vi "MenySMO.vi"() -> ()   [LabVIEW 2018]
uses:
  <vilib>/addons/database/Connection.llb/Conn ObjectReference.ctl
  <vilib>/addons/database/Connection.llb/DB Tools Open Connec (Path).vi
  <vilib>/addons/database/NI_Database_API.lvlib
panel:
  out "Menu Home":bool
  out "Menu Suma":bool
  out "Menu Precios":bool
  in  "Menu":enum32{"Venta", "Precios", "Precios 2"}(tab)
  in  "Guardar Orden":bool
  in  "Reiniciar Orden":bool
  out "Cambio (Pesos)":dbl
  out "TOTAL":dbl
  in  "Orden":string
  in  "PAGO CON:":dbl
  out "Dolares":bool
  out "Tarjeta":bool
  out "Pesos":bool=TRUE
  out "Producto 6":bool
  out "Producto 5":bool
  out "Producto 4":bool
  out "Producto 3":bool
  out "Producto 2":bool
  out "Producto 1":bool
  in  "Tipo de Cambio Dolares":dbl=19.0
  in  "Precio ARROZ CON LECHE":dbl=30.0
  in  "Precio BANDERILLA":dbl=50.0
  in  "Precio PAPAS LOCAS":dbl=50.0
  in  "Precio GOMITAS":dbl=35.0
  in  "Precio PAY DE QUESO":dbl=35.0
  in  "Precio PAN DE MUERTO":dbl=70.0
  in  "Productos":i32(listbox)
  in  "Ventas":i32(listbox)
  in  "OK":bool
  # "ORDEN"
  # "TIPO DE PAGO"
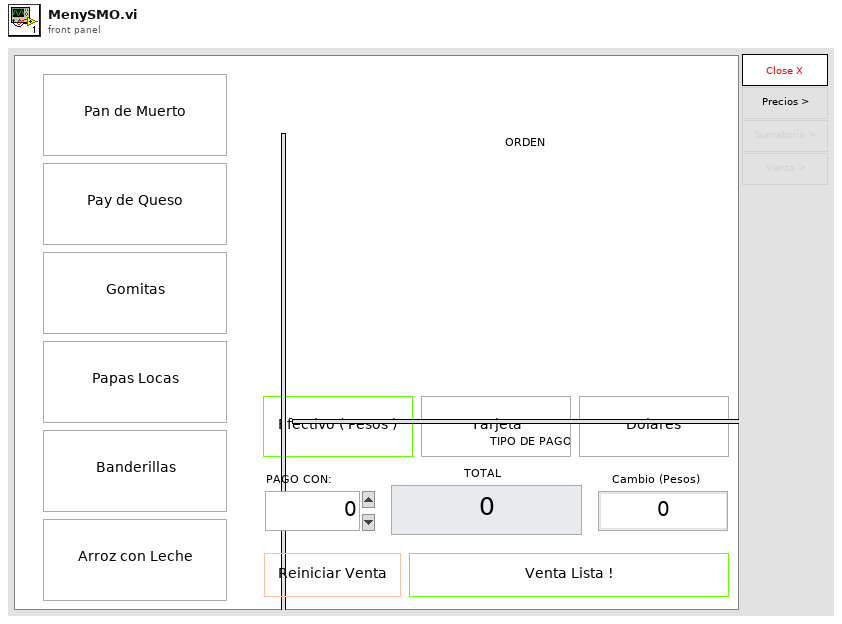
[diagram p1: front panel]
types:
  T1 = enum32{"Invalid", "Standard", "Closed", "Hidden", "Minimized", "Maximized"}
  T2 = enum32{"invalid app kind", "Development System", "Run Time System", "Student Edition", "Embedded LabVIEW", "Evaluation", "Custom"}
  T3 = typedef "NI_Database_API.lvlib/Conn ObjectReference.ctl" = refnum<k1>
  T4 = cluster{"Core":cluster{"Current VI Reference":refnum<vi>, "Close Panel on Exit?":bool}, "Application Directory":path, "Config ADCS":path, "DB":T3, "Productos":string[][], "Ventas":string[][]}
  T5 = cluster{"Current VI Reference":refnum<vi>, "Close Panel on Exit?":bool}
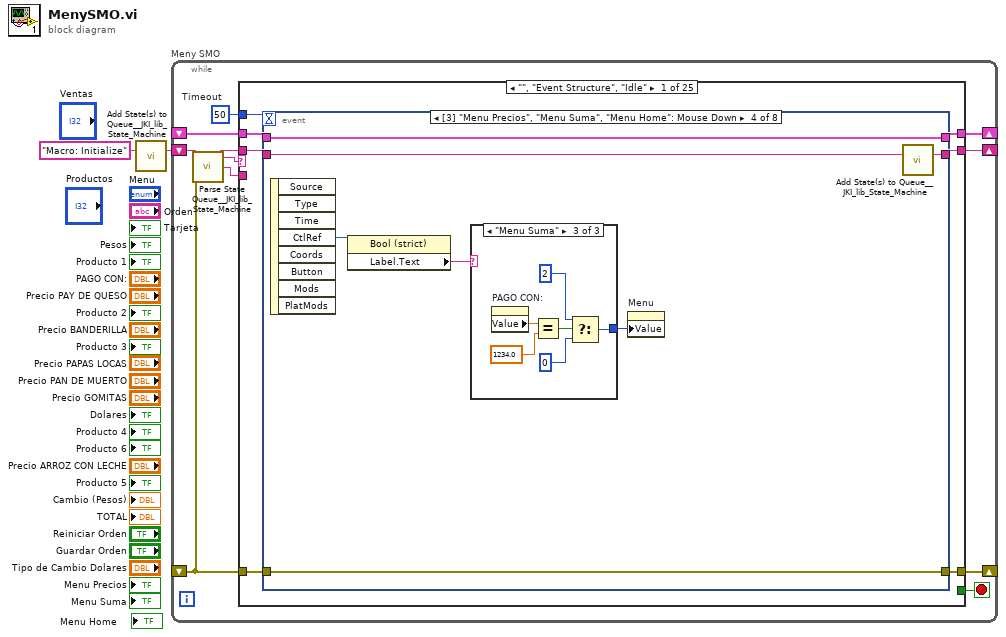
[diagram p0: block diagram]
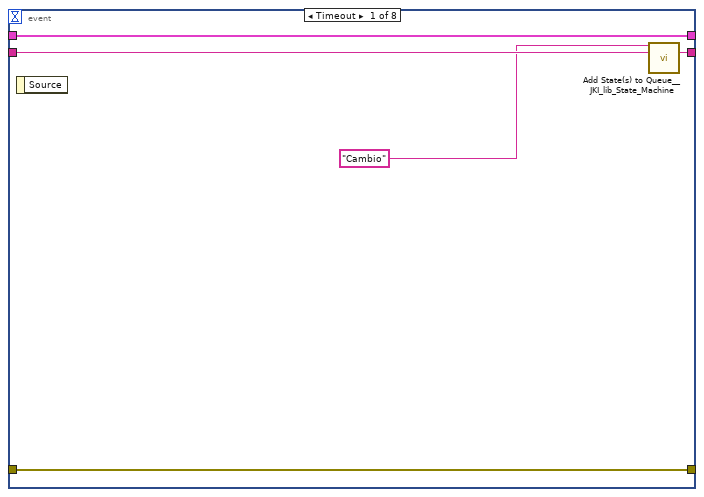
[diagram p2: hidden frame]
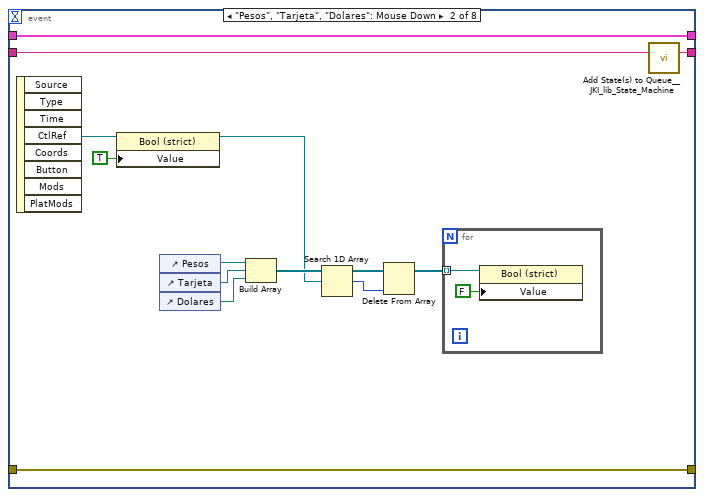
[diagram p3: hidden frame]
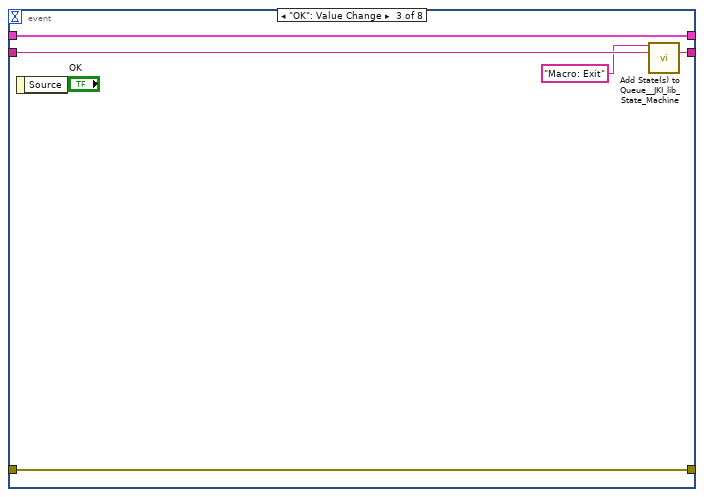
[diagram p4: hidden frame]
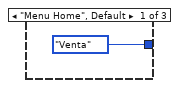
[diagram p5: hidden frame]
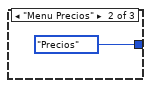
[diagram p6: hidden frame]
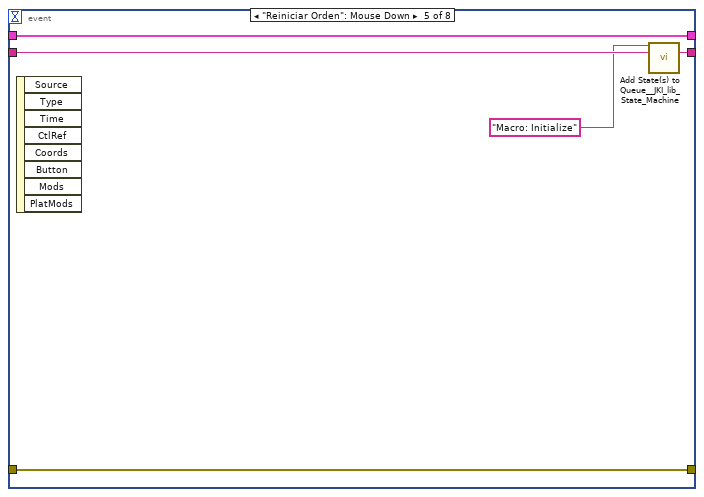
[diagram p7: hidden frame]
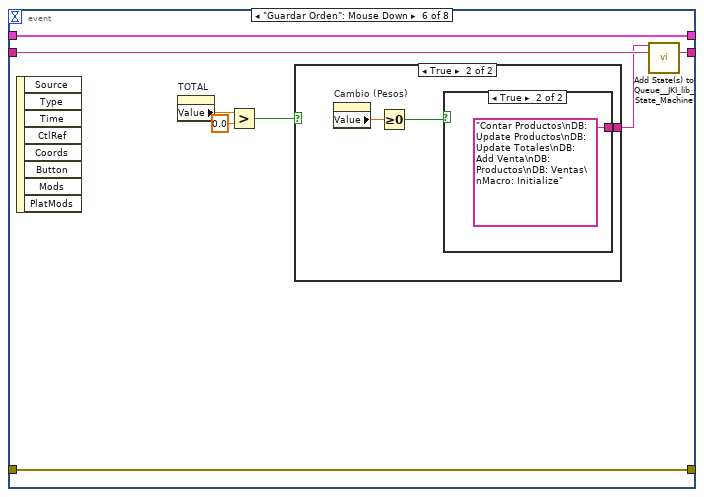
[diagram p8: hidden frame]
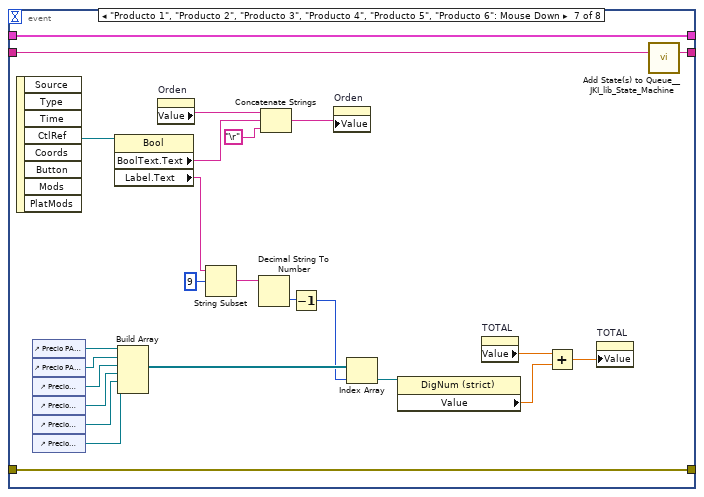
[diagram p11: hidden frame]
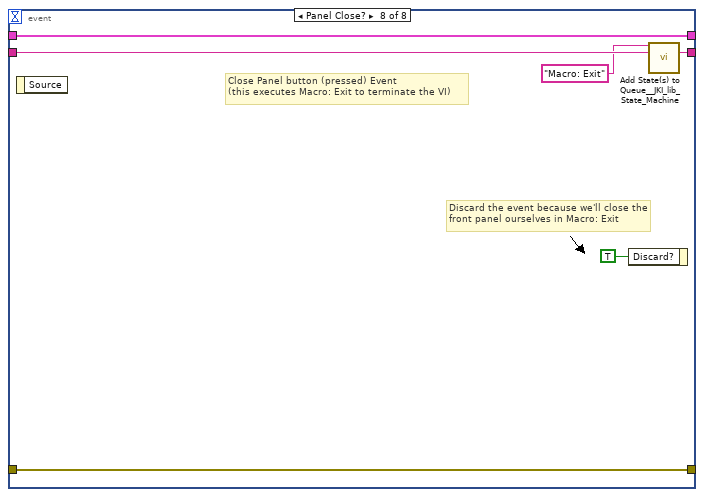
[diagram p12: hidden frame]
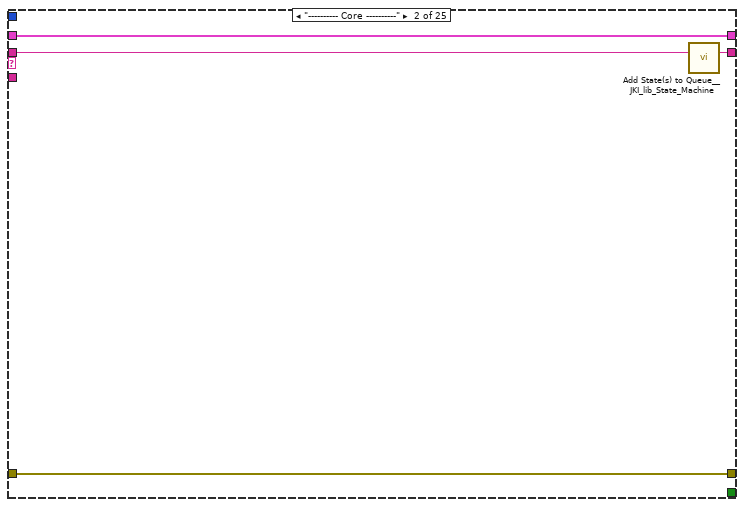
[diagram p13: hidden frame]
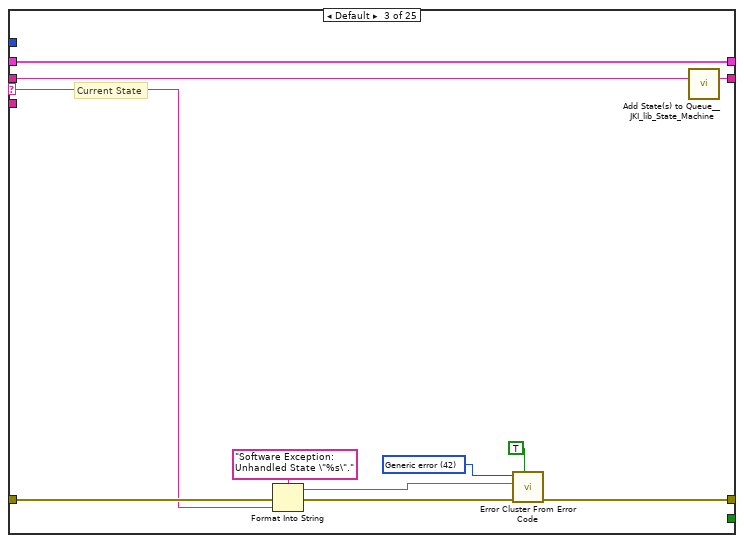
[diagram p14: hidden frame]
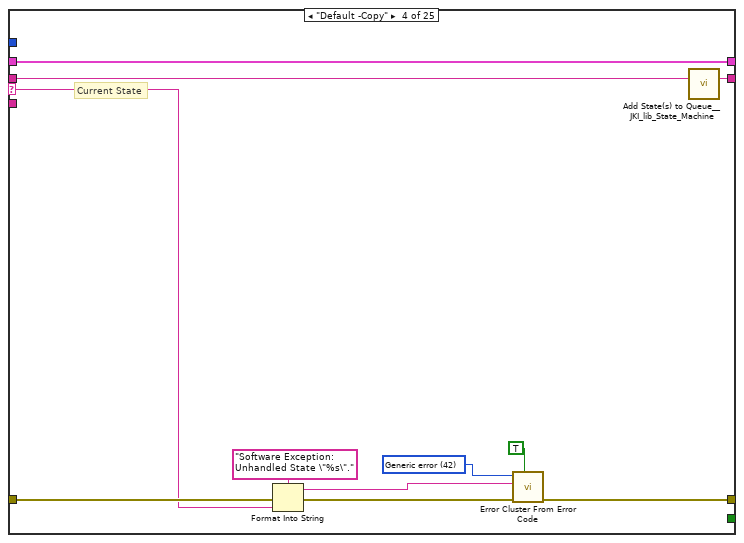
[diagram p15: hidden frame]
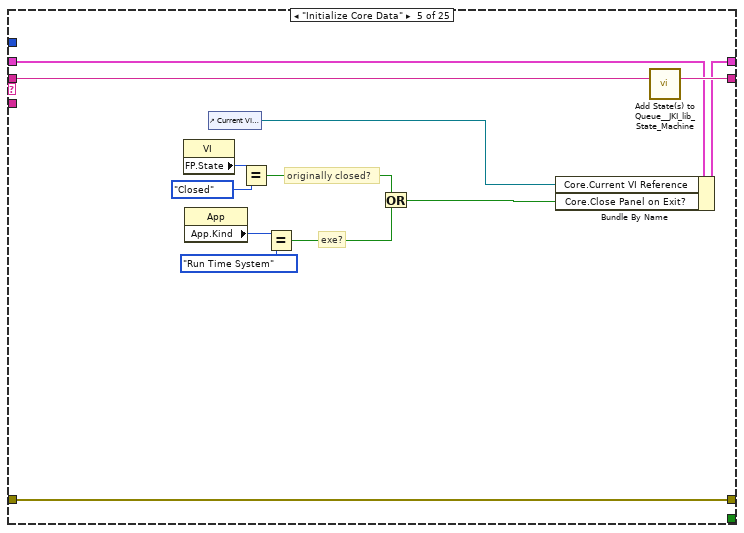
[diagram p16: hidden frame]
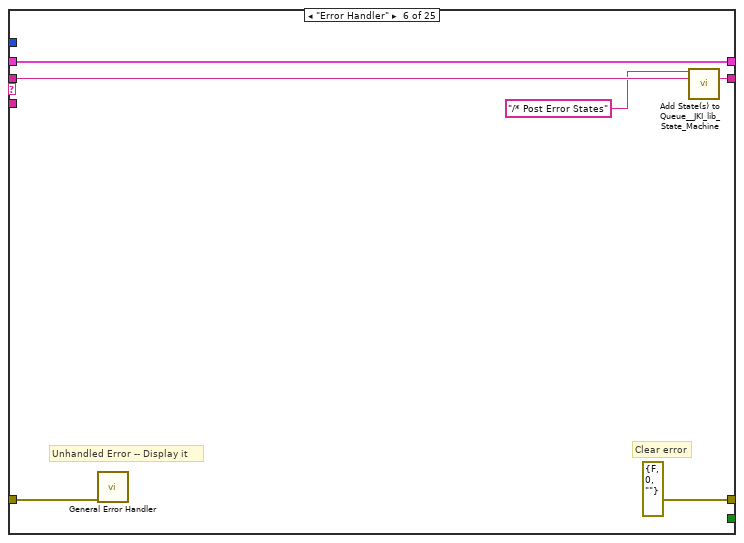
[diagram p17: hidden frame]
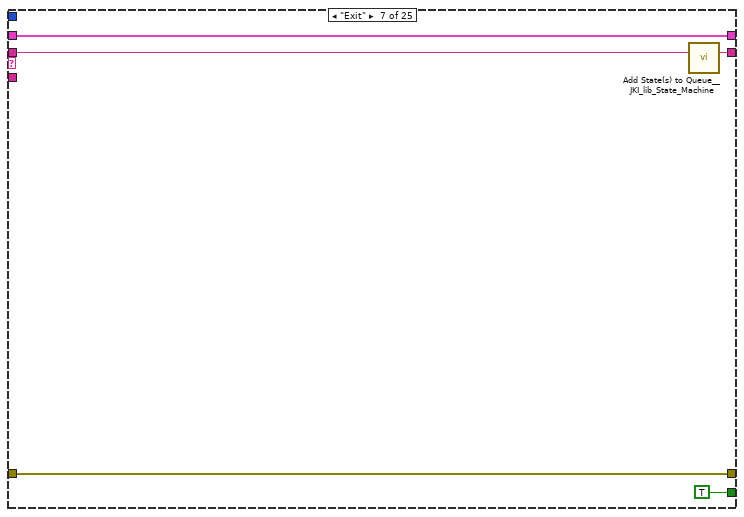
[diagram p18: hidden frame]
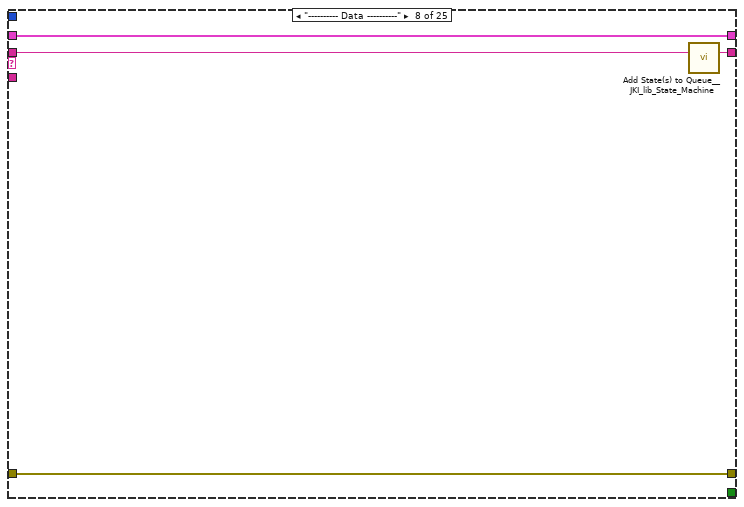
[diagram p19: hidden frame]
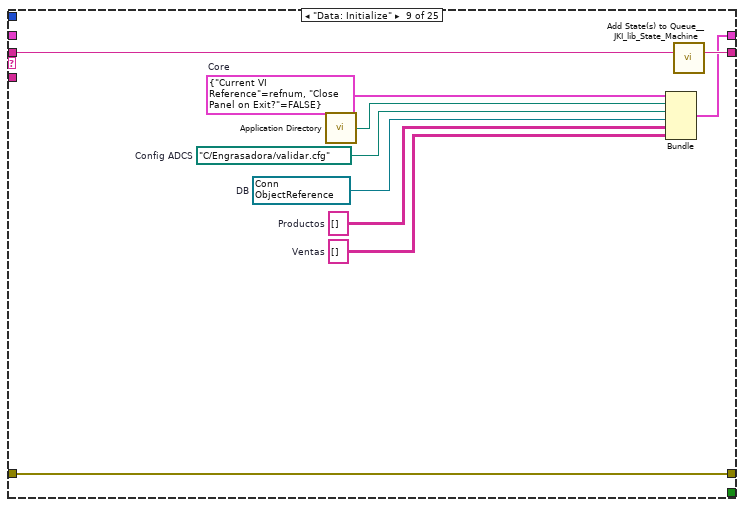
[diagram p20: hidden frame]
diagram:
  n1 = call <vilib>:"Add State(s) to Queue__JKI_lib_State_Machine.vi"("State(s) in (\"\")"="Macro: Initialize") -> ("States Out"=w2:string)  [unwired: 14 in]
  n2 = while "Meny SMO" {
    shift-right: [w6] -> _
    shift-left: _ -> [w5]
    shift-right: [w9] -> _
    shift-left: _ -> [w3]
    shift-right: [w8] -> _
    shift-left: w2 -> [w10]
    stop <- w7 stop-if-true
    w4 = 50  # Timeout
    n3 = call <vilib>:"Parse State Queue__JKI_lib_State_Machine.vi"("State Queue"=w10, "Error In (no error)"=w3) -> ("Remaining States"=w12:string, "Current State"=w13:string, "Arguments"=w11:string)  [unwired: 11 in]
    n4 = case shown="\"\", \"Event Structure\", \"Idle\"" w13 {
      selector: w13 -> [_ _ w113 w124 _ _ _ _ _ _ _ _ _ _ _ _ _ _ _ _ _ _ _ _ _]
      tunnel: w12 -> [w20 w112 w117 w128 w147 w153 w158 w162 w172 w178 w182 w186 w192 w203 w272 w286 w297 w319 w341 w353 w370 w408 w437 w456 w461]
      tunnel: w11 -> [_ _ _ _ _ _ _ _ _ _ _ _ w187 w197 _ _ _ _ _ _ _ _ _ _ _]
      tunnel: w5 -> [w18 w109 w115 w126 w140 w150 w156 w159 _ w173 w179 w184 w190 w199 w269 w283 w294 w306 w334 w349 w368 w406 w433 w452 w458]
      tunnel: [w17 w110 w119 w130 w144 errorcluster {"status"=FALSE, "code"=0, "source"=""} ("error out") w155 w160 w169 w174 w180 w183 w188 w200 w270 w284 w295 w317 w335 w350 w354 w392 w434 w453 w459] -> w9
      tunnel: w3 -> [w16 w110 w118 w129 w144 w149 w155 w160 w169 w175 w180 w183 w189 w201 w270 w284 w295 w317 w336 w351 w355 w393 w435 w454 w459]
      tunnel: [w19 w111 w116 w127 w146 w152 w157 w161 w171 w177 w181 w185 w191 w202 w271 w285 w296 w318 w340 w352 w369 w407 w436 w455 w460] -> w8
      tunnel: [_ _ _ _ _ _ TRUE _ _ _ _ _ _ _ _ _ _ _ _ _ _ _ _ _ _] -> w7
      tunnel: [w15 w109 w115 w126 w145 w150 w156 w159 w170 w173 w179 w184 w190 w199 w269 w283 w294 w298 w333 w348 w367 w405 w432 w451 w458] -> w6
      tunnel: w4 -> [w14 _ _ _ _ _ _ _ _ _ _ _ _ _ _ _ _ _ _ _ _ _ _ _ _]
      frame "", "Event Structure", "Idle" {
        n5 = event shown="[3] \"Menu Precios\", \"Menu Suma\", \"Menu Home\": Mouse Down" {
          selector: _ -> [_ _ _ _ _ _ _ _]
          dyn-events: _ -> [_ _ _ _ _ _ _ _]
          timeout: w14 -> [_ _ _ _ _ _ _ _]
          tunnel: w20 -> [w25 w38 w45 w52 w65 w73 w102 w108]
          tunnel: [w24 w37 w44 w51 w64 w72 w101 w107] -> w19
          tunnel: w18 -> [w22 w35 w42 w49 w62 w70 w99 w105]
          tunnel: [w23 w36 w43 w50 w63 w71 w100 w106] -> w17
          tunnel: w16 -> [w23 w36 w43 w50 w63 w71 w100 w106]
          tunnel: [w22 w35 w42 w49 w62 w70 w99 w105] -> w15
          event Timeout {
            n6 = event-data() -> ()  [unwired: 1 in, 1 out]
            n7 = call <vilib>:"Add State(s) to Queue__JKI_lib_State_Machine.vi"("State(s) in Front (\"\")"="Cambio" ("State(s) in Front (\"\")"), "State(s) in (\"\")"=w25) -> ("States Out"=w24:string)  [unwired: 13 in]
          }
          event "Pesos", "Tarjeta", "Dolares": Mouse Down {
            n8 = event-data() -> ("CtlRef"=w31:refnum<vi>)  [unwired: 1 in, 7 out]
            n9 = property class="Bool (strict)"(reference=w31, "Value"=TRUE) -> (reference out=w28:refnum<vi>)  [unwired: 1 in, 1 out]
            n10 = control-ref of="Pesos"() -> (w34:refnum<vi>)
            n11 = control-ref of="Tarjeta"() -> (w33:refnum<vi>)
            n12 = control-ref of="Dolares"() -> (w32:refnum<vi>)
            n13 = Build Array(w34, w33, w32) -> (w29:refnum<vi>[])
            n14 = Search 1D Array(1D array=w29, element=w28) -> (index of element=w27:i32)  [unwired: 1 in]
            n15 = Delete From Array(array=w29, index=w27) -> (array with subset deleted=w26:refnum<vi>[])  [unwired: 1 in, 1 out]
            n16 = for {
              tunnel: w26 -> [w39] mode=indexing
              n17 = property class="Bool (strict)"(reference=w39, "Value"=FALSE) -> ()  [unwired: 1 in, 2 out]
            }
            n18 = call <vilib>:"Add State(s) to Queue__JKI_lib_State_Machine.vi"("State(s) in (\"\")"=w38) -> ("States Out"=w37:string)  [unwired: 14 in]
          }
          event "OK": Value Change {
            n19 = event-data() -> ()  [unwired: 1 in, 1 out]
            n20 = call <vilib>:"Add State(s) to Queue__JKI_lib_State_Machine.vi"("State(s) in Front (\"\")"="Macro: Exit", "State(s) in (\"\")"=w45) -> ("States Out"=w44:string)  [unwired: 13 in]
          }
          event "Menu Precios", "Menu Suma", "Menu Home": Mouse Down {
            n21 = event-data() -> ("CtlRef"=w47:refnum<vi>)  [unwired: 1 in, 7 out]
            n22 = property class="Bool (strict)"(reference=w47) -> ("Label.Text"=w46:string)  [unwired: 1 in, 2 out]
            n23 = case shown="\"Menu Suma\"" w46 {
              tunnel: [enum32{"Venta", "Precios"}."Venta" ("Menu") enum32{"Venta", "Precios"}."Precios" ("Menu") w55] -> w48
              frame "Menu Home", Default {
              }
              frame "Menu Precios" {
              }
              frame "Menu Suma" {
                n24 = property on="PAGO CON:" class="DigNum (strict)"() -> ("Value"=w60:dbl)  [unwired: 2 in, 2 out]
                n25 = Equal?(x=w60, y=1234.0) -> (x = y?=w58:bool)
                n26 = Select(t=2, s=w58, f=0) -> (s? t:f=w55:i32)
              }
            }
            n27 = property on="Menu" class="TabCtl (strict)"("Value"=w48) -> ()  [unwired: 2 in, 2 out]
            n28 = call <vilib>:"Add State(s) to Queue__JKI_lib_State_Machine.vi"("State(s) in (\"\")"=w52) -> ("States Out"=w51:string)  [unwired: 14 in]
          }
          event "Reiniciar Orden": Mouse Down {
            n29 = event-data() -> ()  [unwired: 1 in, 8 out]
            n30 = call <vilib>:"Add State(s) to Queue__JKI_lib_State_Machine.vi"("State(s) in Front (\"\")"="Macro: Initialize", "State(s) in (\"\")"=w65) -> ("States Out"=w64:string)  [unwired: 13 in]
          }
          event "Guardar Orden": Mouse Down {
            n31 = event-data() -> ()  [unwired: 1 in, 8 out]
            n32 = property on="TOTAL" class="DigNum (strict)"() -> ("Value"=w68:dbl)  [unwired: 2 in, 2 out]
            n33 = Greater?(x=w68, y=0.0) -> (0:w66:bool)
            n34 = case shown="True" w66 {
              tunnel: [_ w76] -> w69
              frame False {
              }
              frame True {
                n35 = property on="Cambio (Pesos)" class="DigNum (strict)"() -> ("Value"=w75:dbl)  [unwired: 2 in, 2 out]
                n36 = Greater Or Equal To 0?(x=w75) -> (x >= 0?=w74:bool)
                n37 = case shown="True" w74 {
                  tunnel: [_ "Contar Productos\nDB: Update Productos\nDB: Update Totales\nDB: Add Venta\nDB: Productos\nDB: Ventas\nMacro: Initialize"] -> w76
                  frame False {
                  }
                  frame True {
                  }
                }
              }
            }
            n38 = call <vilib>:"Add State(s) to Queue__JKI_lib_State_Machine.vi"("State(s) in Front (\"\")"=w69, "State(s) in (\"\")"=w73) -> ("States Out"=w72:string)  [unwired: 13 in]
          }
          event "Producto 1", "Producto 2", "Producto 3", "Producto 4", "Producto 5", "Producto 6": Mouse Down {
            n39 = event-data() -> ("CtlRef"=w98:refnum<vi>)  [unwired: 1 in, 7 out]
            n40 = control-ref of="Precio PAN DE MUERTO"() -> (w97:refnum<vi>)
            n41 = control-ref of="Precio PAY DE QUESO"() -> (w96:refnum<vi>)
            n42 = control-ref of="Precio GOMITAS"() -> (w95:refnum<vi>)
            n43 = control-ref of="Precio PAPAS LOCAS"() -> (w94:refnum<vi>)
            n44 = control-ref of="Precio BANDERILLA"() -> (w93:refnum<vi>)
            n45 = control-ref of="Precio ARROZ CON LECHE"() -> (w92:refnum<vi>)
            n46 = property class="Bool"(reference=w98) -> ("BoolText.Text"=w80:string, "Label.Text"=w90:string)  [unwired: 1 in, 2 out]
            n47 = Build Array(w97, w96, w95, w94, w93, w92) -> (w91:refnum<vi>[])
            n48 = property on="Orden" class="Str"() -> ("Value"=w81:string)  [unwired: 2 in, 2 out]
            n49 = String Subset(string=w90, offset (0)=9) -> (substring=w88:string)  [unwired: 1 in]
            n50 = Decimal String To Number(string=w88) -> (number=w87:i32)  [unwired: 2 in, 1 out]
            n51 = Concatenate Strings(w81, w80, "\r") -> (w78:string)
            n52 = Decrement(x=w87) -> (x-1=w86:i32)
            n53 = property on="Orden" class="Str"("Value"=w78) -> ()  [unwired: 2 in, 2 out]
            n54 = Index Array(array=w91, index=w86) -> (element=w85:refnum<vi>)
            n55 = property class="DigNum (strict)"(reference=w85) -> ("Value"=w83:dbl)  [unwired: 1 in, 2 out]
            n56 = property on="TOTAL" class="DigNum (strict)"() -> ("Value"=w84:dbl)  [unwired: 2 in, 2 out]
            n57 = Add(x=w84, y=w83) -> (x+y=w82:dbl)
            n58 = property on="TOTAL" class="DigNum (strict)"("Value"=w82) -> ()  [unwired: 2 in, 2 out]
            n59 = call <vilib>:"Add State(s) to Queue__JKI_lib_State_Machine.vi"("State(s) in (\"\")"=w102) -> ("States Out"=w101:string)  [unwired: 14 in]
          }
          event Panel Close? {
            # "Discard the event because we'll close the front panel ourselves in Macro: Exit"
            # "Close Panel button (pressed) Event\n(this executes Macro: Exit to terminate the VI)"
            n60 = event-data() -> ()  [unwired: 1 in, 1 out]
            n61 = event-data("Discard?"=TRUE) -> ()  [unwired: 1 in, 1 out]
            n62 = call <vilib>:"Add State(s) to Queue__JKI_lib_State_Machine.vi"("State(s) in Front (\"\")"="Macro: Exit", "State(s) in (\"\")"=w108) -> ("States Out"=w107:string)  [unwired: 13 in]
          }
        }
      }
      frame "---------- Core ----------" {
        n63 = call <vilib>:"Add State(s) to Queue__JKI_lib_State_Machine.vi"("State(s) in (\"\")"=w112) -> ("States Out"=w111:string)  [unwired: 14 in]
      }
      frame Default {
        w122 = 42 items=["No error", "Argument error", "Memory is full", "Out of zone", "End of file", "File already open", "Generic file I/O error", "File not found", "File permission error", "Disk is full", "Duplicate path", "Too many files open", "System feature not enabled", "Resource file not found", "Cannot add resource", "Resource not found", "Image not found", "Image memory error", "Pen does not exist", "Config type invalid", "Config token not found", "Config parse error", "Config memory error", "Bad external code format", "Bad external code offset", "External code not present", "Null window", "Destroy window error", "Null menu", "Print aborted", "Bad print record", "Print driver error", "Windows error during printing", "Memory error during printing", "Print dialog error", "Generic print error", "Invalid device refnum", "Device not found", "Device parameter error", "Device unit error", "Cannot open device", "Device call aborted", "Generic error", "Cancelled by user", "Object ID too low", "Object ID too high", "Object not in heap", "Unknown heap", "Unknown object (invalid DefProc)", "Unknown object (DefProc not in table)", "Message out of range", "Invalid (null) method", "Unknown message", "Manager call not supported", "Bad address", "Network operation in progress", "Network operation timed out", "Connection is busy", "Network attribute not supported", "Network error", "Address in use", "System out of memory", "Connection aborted", "Connection refused", "Not connected", "Already connected", "Connection closed", "Initialization error (interapplication manager)", "Bad occurrence", "Wait on unbound occurrence handler", "Occurrence queue overflow", "Datalog type conflict", "Unused", "Unrecognized type (interapplication manager)", "Memory corrupt", "Failed to make temporary DLL", "Old CIN version", "Drag socket not found", "Failed to load drop-object", "Failed to register OLE object", "Failed to release OLE object", "Format specifier type mismatch", "Unknown format specifier", "Too few format specifiers", "Too many format specifiers", "Scan failed", "Newer CIN version", "Error converting to variant", "Runtime menu error", "Password tampered", "Variant attribute not found", "Incompatible variant data type", "Event data is not available", "Event Store is not present", "Occurrence is not found", "Event Queue is not created", "Event info is not available", "Refnum passed is NULL", "Error retrieving Class GUID", "Error retrieving CoClass GUID", "Error retrieving TypeLib GUID.", "Bad built application magic bytes.", "Specific driver is different from the specific driver associated with the Logical Name.", "There is no session opened to the class driver.", "Max Error", "MAX - Error with config objects", "MAX - Error loading configuration", "MAX - Group not supported"]
        # "Current State"
        n64 = Format Into String(format string="Software Exception: Unhandled State \"%s\"." ("message"), error in=w118, w113) -> (resulting string=w121:string, error out=w120:errorcluster)  [unwired: 1 in]
        n65 = call <vilib>:"Error Cluster From Error Code.vi"("show call chain? (False)"=TRUE, "error in (no error)"=w120, "error message (\"\")"=w121, "error code (0)"=w122) -> ("error out"=w119:errorcluster)  [unwired: 5 in]
        n66 = call <vilib>:"Add State(s) to Queue__JKI_lib_State_Machine.vi"("State(s) in (\"\")"=w117) -> ("States Out"=w116:string)  [unwired: 14 in]
      }
      frame "Default -Copy" {
        w133 = 42 items=["No error", "Argument error", "Memory is full", "Out of zone", "End of file", "File already open", "Generic file I/O error", "File not found", "File permission error", "Disk is full", "Duplicate path", "Too many files open", "System feature not enabled", "Resource file not found", "Cannot add resource", "Resource not found", "Image not found", "Image memory error", "Pen does not exist", "Config type invalid", "Config token not found", "Config parse error", "Config memory error", "Bad external code format", "Bad external code offset", "External code not present", "Null window", "Destroy window error", "Null menu", "Print aborted", "Bad print record", "Print driver error", "Windows error during printing", "Memory error during printing", "Print dialog error", "Generic print error", "Invalid device refnum", "Device not found", "Device parameter error", "Device unit error", "Cannot open device", "Device call aborted", "Generic error", "Cancelled by user", "Object ID too low", "Object ID too high", "Object not in heap", "Unknown heap", "Unknown object (invalid DefProc)", "Unknown object (DefProc not in table)", "Message out of range", "Invalid (null) method", "Unknown message", "Manager call not supported", "Bad address", "Network operation in progress", "Network operation timed out", "Connection is busy", "Network attribute not supported", "Network error", "Address in use", "System out of memory", "Connection aborted", "Connection refused", "Not connected", "Already connected", "Connection closed", "Initialization error (interapplication manager)", "Bad occurrence", "Wait on unbound occurrence handler", "Occurrence queue overflow", "Datalog type conflict", "Unused", "Unrecognized type (interapplication manager)", "Memory corrupt", "Failed to make temporary DLL", "Old CIN version", "Drag socket not found", "Failed to load drop-object", "Failed to register OLE object", "Failed to release OLE object", "Format specifier type mismatch", "Unknown format specifier", "Too few format specifiers", "Too many format specifiers", "Scan failed", "Newer CIN version", "Error converting to variant", "Runtime menu error", "Password tampered", "Variant attribute not found", "Incompatible variant data type", "Event data is not available", "Event Store is not present", "Occurrence is not found", "Event Queue is not created", "Event info is not available", "Refnum passed is NULL", "Error retrieving Class GUID", "Error retrieving CoClass GUID", "Error retrieving TypeLib GUID.", "Bad built application magic bytes.", "Specific driver is different from the specific driver associated with the Logical Name.", "There is no session opened to the class driver.", "Max Error", "MAX - Error with config objects", "MAX - Error loading configuration", "MAX - Group not supported"]
        # "Current State"
        n67 = Format Into String(format string="Software Exception: Unhandled State \"%s\"." ("message"), error in=w129, w124) -> (resulting string=w132:string, error out=w131:errorcluster)  [unwired: 1 in]
        n68 = call <vilib>:"Error Cluster From Error Code.vi"("show call chain? (False)"=TRUE, "error in (no error)"=w131, "error message (\"\")"=w132, "error code (0)"=w133) -> ("error out"=w130:errorcluster)  [unwired: 5 in]
        n69 = call <vilib>:"Add State(s) to Queue__JKI_lib_State_Machine.vi"("State(s) in (\"\")"=w128) -> ("States Out"=w127:string)  [unwired: 14 in]
      }
      frame "Initialize Core Data" {
        # "originally closed?"
        # "exe?"
        n70 = property class="VI"() -> ("FP.State"=w137:T1)  [unwired: 2 in, 2 out]
        n71 = property class="App"() -> ("App.Kind"=w143:T2)  [unwired: 2 in, 2 out]
        n72 = control-ref of="Current VI Reference"() -> (w138:refnum<vi>)
        n73 = Equal?(x=w137, y=T1."Closed" ("Front Panel Window:State")) -> (x = y?=w135:bool)
        n74 = Equal?(x=w143, y=T2."Run Time System" ("Application:Kind")) -> (x = y?=w141:bool)
        n75 = Or(x=w135, y=w141) -> (x .or. y?=w139:bool)
        n76 = Bundle By Name(cluster=w140, "Core.Current VI Reference"=w138, "Core.Close Panel on Exit?"=w139) -> (w145:T4)
        n77 = call <vilib>:"Add State(s) to Queue__JKI_lib_State_Machine.vi"("State(s) in (\"\")"=w147) -> ("States Out"=w146:string)  [unwired: 14 in]
      }
      frame "Error Handler" {
        # "Unhandled Error -- Display it"
        # "Clear error"
        n78 = call <vilib>:"General Error Handler.vi"("error in (no error)"=w149) -> ()  [unwired: 10 in, 5 out]
        n79 = call <vilib>:"Add State(s) to Queue__JKI_lib_State_Machine.vi"("State(s) in Front (\"\")"="/* Post Error States", "State(s) in (\"\")"=w153) -> ("States Out"=w152:string)  [unwired: 13 in]
      }
      frame "Exit" {
        n80 = call <vilib>:"Add State(s) to Queue__JKI_lib_State_Machine.vi"("State(s) in (\"\")"=w158) -> ("States Out"=w157:string)  [unwired: 14 in]
      }
      frame "---------- Data ----------" {
        n81 = call <vilib>:"Add State(s) to Queue__JKI_lib_State_Machine.vi"("State(s) in (\"\")"=w162) -> ("States Out"=w161:string)  [unwired: 14 in]
      }
      frame "Data: Initialize" {
        w163 = string[][] []  # Ventas
        w164 = string[][] []  # Productos
        w165 = T3 refnum items=["Connection"]  # DB
        w166 = path "C:/Engrasadora/validar.cfg"  # Config ADCS
        w168 = T5 {"Current VI Reference"=refnum, "Close Panel on Exit?"=FALSE}  # Core
        n82 = call <vilib>:"Application Directory.vi"() -> ("Application Directory"=w167:path)
        n83 = Bundle("Core"=w168, "Application Directory"=w167, "Config ADCS"=w166, "DB"=w165, "Productos"=w164, "Ventas"=w163) -> (w170:T4)  [unwired: 1 in]
        n84 = call <vilib>:"Add State(s) to Queue__JKI_lib_State_Machine.vi"("State(s) in (\"\")"=w172) -> ("States Out"=w171:string)  [unwired: 14 in]
      }
      frame "Data: Cleanup" {
        n85 = Unbundle By Name(w173) -> ("Core.Current VI Reference"=w176:refnum<vi>)
        n86 = Close Reference(reference=w176, error in (no error)=w175) -> (error out=w174:errorcluster)
        n87 = call <vilib>:"Add State(s) to Queue__JKI_lib_State_Machine.vi"("State(s) in (\"\")"=w178) -> ("States Out"=w177:string)  [unwired: 14 in]
      }
      frame "---------- UI ----------" {
        n88 = call <vilib>:"Add State(s) to Queue__JKI_lib_State_Machine.vi"("State(s) in (\"\")"=w182) -> ("States Out"=w181:string)  [unwired: 14 in]
      }
      frame "UI: Initialize" {
        n89 = call <vilib>:"Add State(s) to Queue__JKI_lib_State_Machine.vi"("State(s) in (\"\")"=w186) -> ("States Out"=w185:string)  [unwired: 14 in]
      }
      frame "UI: Cursor Set" {
        # "Argument"
        n90 = case shown="\"Idle\", Default" w187 {
          tunnel: w189 -> [w194 w196]
          tunnel: [w193 w195] -> w188
          frame "Idle", Default {
            n91 = call <vilib>:"Unset Busy.vi"("error in (no error)"=w194) -> ("error out"=w193:errorcluster)  [unwired: 10 in]
          }
          frame "Busy" {
            n92 = call <vilib>:"Set Busy.vi"("error in (no error)"=w196) -> ("error out"=w195:errorcluster)  [unwired: 9 in, 1 out]
          }
        }
        n93 = call <vilib>:"Add State(s) to Queue__JKI_lib_State_Machine.vi"("State(s) in (\"\")"=w192) -> ("States Out"=w191:string)  [unwired: 14 in]
      }
      frame "UI: Front Panel State" {
        # "Argument"
        n94 = Unbundle By Name(w199) -> ("Core.Current VI Reference"=w198:refnum<vi>)
        n95 = case shown="\"Minimize\", \"Minimized\"" w197 {
          tunnel: w201 -> [w209 w224 w235 w248 w261]
          tunnel: [w211 w225 w237 w250 w263] -> w200
          tunnel: w198 -> [w210 w222 w236 w249 w262]
          frame "Open", "Standard", Default {
            w204 = T1."Standard" ("State")
            n96 = property class="VI"(reference=w210, error in=w209) -> (reference out=w207:refnum<vi>, error out=w208:errorcluster, "FP.State"=w206:T1)
            n97 = Not Equal?(x=w206, y=w204) -> (x != y?=w205:bool)
            n98 = case shown="True" w205 {
              tunnel: [w215 w217] -> w211
              tunnel: w208 -> [w214 w217]
              tunnel: w207 -> [w213 _]
              tunnel: w204 -> [w212 _]
              frame True {
                n99 = invoke class="VI" method="FP.Open"(reference=w213, error in=w214, "Activate"=TRUE, "State"=w212) -> (error out=w215:errorcluster)  [unwired: 1 in, 4 out]
              }
              frame False {
              }
            }
          }
          frame "Close", "Closed" {
            n100 = property class="VI"(reference=w222, error in=w224) -> (reference out=w221:refnum<vi>, error out=w223:errorcluster, "FP.State"=w219:T1)
            n101 = Not Equal?(x=w219, y=T1."Closed" ("Front Panel Window:State")) -> (x != y?=w218:bool)
            n102 = case shown="True" w218 {
              tunnel: [w226 w229] -> w225
              tunnel: w223 -> [w226 w228]
              tunnel: w221 -> [_ w227]
              frame False {
              }
              frame True {
                n103 = invoke class="VI" method="FP.Close"(reference=w227, error in=w228) -> (error out=w229:errorcluster)  [unwired: 1 in, 2 out]
              }
            }
          }
          frame "Hidden", "Hide" {
            w230 = T1."Hidden" ("State")
            n104 = property class="VI"(reference=w236, error in=w235) -> (reference out=w233:refnum<vi>, error out=w234:errorcluster, "FP.State"=w232:T1)
            n105 = Not Equal?(x=w232, y=w230) -> (x != y?=w231:bool)
            n106 = case shown="True" w231 {
              tunnel: [w241 w242] -> w237
              tunnel: w234 -> [w240 w242]
              tunnel: w233 -> [w239 _]
              tunnel: w230 -> [w238 _]
              frame True {
                n107 = invoke class="VI" method="FP.Open"(reference=w239, error in=w240, "State"=w238) -> (error out=w241:errorcluster)  [unwired: 2 in, 4 out]
              }
              frame False {
              }
            }
          }
          frame "Minimize", "Minimized" {
            w243 = T1."Minimized" ("State")
            n108 = property class="VI"(reference=w249, error in=w248) -> (reference out=w246:refnum<vi>, error out=w247:errorcluster, "FP.State"=w245:T1)
            n109 = Not Equal?(x=w245, y=w243) -> (x != y?=w244:bool)
            n110 = case shown="True" w244 {
              tunnel: [w254 w255] -> w250
              tunnel: w247 -> [w253 w255]
              tunnel: w246 -> [w252 _]
              tunnel: w243 -> [w251 _]
              frame True {
                n111 = invoke class="VI" method="FP.Open"(reference=w252, error in=w253, "State"=w251) -> (error out=w254:errorcluster)  [unwired: 2 in, 4 out]
              }
              frame False {
              }
            }
          }
          frame "Maximize", "Maximized" {
            w256 = T1."Maximized" ("State")
            n112 = property class="VI"(reference=w262, error in=w261) -> (reference out=w259:refnum<vi>, error out=w260:errorcluster, "FP.State"=w258:T1)
            n113 = Not Equal?(x=w258, y=w256) -> (x != y?=w257:bool)
            n114 = case shown="True" w257 {
              tunnel: [w267 w268] -> w263
              tunnel: w260 -> [w266 w268]
              tunnel: w259 -> [w265 _]
              tunnel: w256 -> [w264 _]
              frame True {
                n115 = invoke class="VI" method="FP.Open"(reference=w265, error in=w266, "State"=w264) -> (error out=w267:errorcluster)  [unwired: 2 in, 4 out]
              }
              frame False {
              }
            }
          }
        }
        n116 = call <vilib>:"Add State(s) to Queue__JKI_lib_State_Machine.vi"("State(s) in (\"\")"=w203) -> ("States Out"=w202:string)  [unwired: 14 in]
      }
      frame "---------- Macro ----------" {
        n117 = call <vilib>:"Add State(s) to Queue__JKI_lib_State_Machine.vi"("State(s) in (\"\")"=w272) -> ("States Out"=w271:string)  [unwired: 14 in]
      }
      frame "Macro: Initialize" {
        w282 = "Data: Initialize\nInitialize Core Data\nUI: Initialize\nUI: Front Panel State >> Open\nDB: Init\nDB: Productos\nDB: Ventas"  # Data: Initialize Initialize Core Data UI: Initialize UI: Front Panel State >> Open DB: Init DB: Productos DB: Ventas
        n118 = control-ref of="Dolares"() -> (w276:refnum<vi>)
        n119 = control-ref of="Tarjeta"() -> (w275:refnum<vi>)
        n120 = control-ref of="Pesos"() -> (w274:refnum<vi>)
        n121 = control-ref of="Cambio (Pesos)"() -> (w280:refnum<vi>)
        n122 = control-ref of="PAGO CON:"() -> (w279:refnum<vi>)
        n123 = control-ref of="TOTAL"() -> (w278:refnum<vi>)
        n124 = control-ref of="Orden"() -> (w281:refnum<vi>)
        n125 = property on="Menu" class="TabCtl (strict)"("Value"=enum32{"Venta", "Precios", "Precios 2"}."Venta" ("Menu")) -> ()  [unwired: 2 in, 2 out]
        n126 = Build Array(w281, w280, w279, w278, w276, w275, w274) -> (w277:refnum<vi>[])
        n127 = for {
          tunnel: w277 -> [w287] mode=indexing
          n128 = invoke class="Ctl" method="Reinit To Default"(reference=w287) -> ()  [unwired: 2 in, 3 out]
        }
        n129 = call <vilib>:"Add State(s) to Queue__JKI_lib_State_Machine.vi"("State(s) in Front (\"\")"=w282, "State(s) in (\"\")"=w286) -> ("States Out"=w285:string)  [unwired: 13 in]
      }
      frame "Macro: Exit" {
        n130 = Unbundle By Name(w294) -> ("Core.Close Panel on Exit?"=w293:bool)
        n131 = Select(t="UI: Front Panel State >> Close", s=w293, f="") -> (s? t:f=w290:string)
        n132 = call <vilib>:"Add State(s) to Queue__JKI_lib_State_Machine.vi"("State(s) in (\"\")"=w290, "State(s) at Back (\"\")"="Data: Cleanup\nExit") -> ("States Out"=w288:string)  [unwired: 13 in]
        n133 = call <vilib>:"Add State(s) to Queue__JKI_lib_State_Machine.vi"("State(s) in Front (\"\")"=w288, "State(s) in (\"\")"=w297) -> ("States Out"=w296:string)  [unwired: 13 in]
      }
      frame "Contar Productos" {
        n134 = Unbundle By Name(w306) -> ("Productos"=w307:string[][])
        n135 = control-ref of="Producto 1"() -> (w316:refnum<vi>)
        n136 = control-ref of="Producto 2"() -> (w315:refnum<vi>)
        n137 = control-ref of="Producto 3"() -> (w314:refnum<vi>)
        n138 = control-ref of="Producto 4"() -> (w313:refnum<vi>)
        n139 = control-ref of="Producto 5"() -> (w312:refnum<vi>)
        n140 = control-ref of="Producto 6"() -> (w311:refnum<vi>)
        n141 = Index Array(array=w307, index (row)=0) -> (element=w308:string[])  [unwired: 1 in]
        n142 = Build Array(w316, w315, w314, w313, w312, w311) -> (w310:refnum<vi>[])
        n143 = for {
          tunnel: w310 -> [w329] mode=indexing
          tunnel: w308 -> [w326]
          tunnel: w307 -> [_]
          tunnel: [w320] -> w302 mode=indexing
          i -> [w327]
          n144 = property class="Bool"(reference=w329) -> ("BoolText.Text"=w328:string)  [unwired: 1 in, 2 out]
          n145 = Increment(x=w327) -> (x+1=w325:i32)
          n146 = property on="Orden" class="Str"() -> ("Value"=w331:string)  [unwired: 2 in, 2 out]
          n147 = Index Array(array=w326, index=w325) -> (element=w324:string)
          n148 = Search and Replace String(replace all?=TRUE ("replace all? (F)"), input string=w331, search string=w328, replace string=w328) -> (number of replacements=w323:i32)  [unwired: 4 in, 3 out]
          n149 = Decimal String To Number(string=w324) -> (number=w322:i32)  [unwired: 2 in, 1 out]
          n150 = Add(x=w323, y=w322) -> (x+y=w321:i32)
          n151 = Number To Decimal String(number=w321) -> (decimal integer string=w320:string)  [unwired: 1 in]
        }
        n152 = Unbundle By Name(w306) -> ("Productos"=w305:string[][])
        n153 = Insert Into Array(array=string[] ["1"], index=1, new element=w302) -> (w299:string[])
        n154 = Replace Array Subset(array=w305, new element=w299, index (row)=0) -> (w304:string[][])  [unwired: 1 in]
        n155 = Bundle By Name(cluster=w306, "Productos"=w304) -> (w298:T4)
        n156 = call <vilib>:"Add State(s) to Queue__JKI_lib_State_Machine.vi"("State(s) in (\"\")"=w319) -> ("States Out"=w318:string)  [unwired: 14 in]
      }
      frame "DB: Init" {
        n157 = Unbundle By Name(w334) -> ("Application Directory"=w339:path)
        n158 = Build Path(base path=w339, name or relative path="DB\\POS.udl") -> (appended path=w337:path)
        n159 = call-poly <vilib>:"DB Tools Open Connection.vi"("error in (no error)"=w336, "connection information"=w337) -> ("error out"=w335:errorcluster, "connection reference"=w332:T3)  [unwired: 6 in]
        n160 = Bundle By Name(cluster=w334, "DB"=w332) -> (w333:T4)
        n161 = call <vilib>:"Add State(s) to Queue__JKI_lib_State_Machine.vi"("State(s) in (\"\")"=w341) -> ("States Out"=w340:string)  [unwired: 14 in]
      }
      frame "DB: Productos" {
        n162 = Unbundle By Name(w349) -> ("DB"=w346:T3)
        n163 = call <vilib>:"DB Tools Select Data.vi"("error in (no error)"=w351, "table"="Productos", "connection reference"=w346) -> ("error out"=w350:errorcluster, "data"=w344:variant[][], "connection reference out"=w347:T3)  [unwired: 3 in]
        n164 = Variant To Data(type=string[][] [] ("table"), Variant=w344) -> (data=w342:string[][])  [unwired: 1 in, 1 out]
        n165 = Bundle By Name(cluster=w349, "DB"=w347, "Productos"=w342) -> (w348:T4)
        n166 = property on="Productos" class="MCListbox (strict)"("ItemNames"=w342) -> ()  [unwired: 2 in, 2 out]
        n167 = call <vilib>:"Add State(s) to Queue__JKI_lib_State_Machine.vi"("State(s) in (\"\")"=w353) -> ("States Out"=w352:string)  [unwired: 14 in]
      }
      frame "DB: Update Productos" {
        n168 = Unbundle By Name(w368) -> ("Productos"=w366:string[][], "DB"=w362:T3)
        n169 = Build Array("Pan", "Pay", "Gomas", "Papas", "Banderilla", "Arroz") -> (w356:string[])
        n170 = for {
          N: 6 -> [_]
          tunnel: w366 -> [w384]
          shift-right: [w376] -> w361
          shift-left: w362 -> [w377]
          tunnel: w356 -> [w375] mode=indexing
          shift-right: [w371] -> w354
          shift-left: w355 -> [w372]
          i -> [w381]
          n171 = Increment(x=w381) -> (x+1=w382:i32)
          n172 = Build Array(w375) -> (w374:string[])
          n173 = Index Array(array=w384, index (row)=0, index (col)=w382) -> (element=w380:string)
          n174 = Decimal String To Number(string=w380) -> (number=w378:i32)  [unwired: 2 in, 1 out]
          n175 = call <vilib>:"DB Tools Update Data.vi"("condition"="where ID = 2", "data"=w378, "error in (no error)"=w372, "columns"=w374, "table"="Productos", "connection reference"=w377) -> ("error out"=w371:errorcluster, "connection reference out"=w376:T3)  [unwired: 4 in]
        }
        n176 = Bundle By Name(cluster=w368, "DB"=w361) -> (w367:T4)
        n177 = call <vilib>:"Add State(s) to Queue__JKI_lib_State_Machine.vi"("State(s) in (\"\")"=w370) -> ("States Out"=w369:string)  [unwired: 14 in]
      }
      frame "DB: Update Totales" {
        n178 = control-ref of="Precio PAN DE MUERTO"() -> (w391:refnum<vi>)
        n179 = control-ref of="Precio PAY DE QUESO"() -> (w390:refnum<vi>)
        n180 = control-ref of="Precio GOMITAS"() -> (w389:refnum<vi>)
        n181 = control-ref of="Precio PAPAS LOCAS"() -> (w388:refnum<vi>)
        n182 = control-ref of="Precio BANDERILLA"() -> (w387:refnum<vi>)
        n183 = control-ref of="Precio ARROZ CON LECHE"() -> (w386:refnum<vi>)
        n184 = Unbundle By Name(w406) -> ("Productos"=w404:string[][], "DB"=w400:T3)
        n185 = Build Array(w391, w390, w389, w388, w387, w386) -> (w385:refnum<vi>[])
        n186 = Build Array("Pan", "Pay", "Gomas", "Papas", "Banderilla", "Arroz") -> (w394:string[])
        n187 = for {
          N: 6 -> [_]
          tunnel: w404 -> [w425]
          shift-right: [w418] -> w399
          shift-left: w400 -> [w419]
          tunnel: w394 -> [w417] mode=indexing
          shift-right: [w413] -> w392
          shift-left: w393 -> [w414]
          tunnel: w385 -> [w412] mode=indexing
          i -> [w422]
          n188 = property class="DigNum (strict)"(reference=w412) -> ("Value"=w411:dbl)  [unwired: 1 in, 2 out]
          n189 = Increment(x=w422) -> (x+1=w423:i32)
          n190 = Build Array(w417) -> (w416:string[])
          n191 = Index Array(array=w425, index (row)=0, index (col)=w423) -> (element=w421:string)
          n192 = Decimal String To Number(string=w421) -> (number=w410:i32)  [unwired: 2 in, 1 out]
          n193 = Multiply(x=w410, y=w411) -> (x*y=w409:dbl)
          n194 = call <vilib>:"DB Tools Update Data.vi"("condition"="where ID = 3", "data"=w409, "error in (no error)"=w414, "columns"=w416, "table"="Productos", "connection reference"=w419) -> ("error out"=w413:errorcluster, "connection reference out"=w418:T3)  [unwired: 4 in]
        }
        n195 = Bundle By Name(cluster=w406, "DB"=w399) -> (w405:T4)
        n196 = call <vilib>:"Add State(s) to Queue__JKI_lib_State_Machine.vi"("State(s) in (\"\")"=w408) -> ("States Out"=w407:string)  [unwired: 14 in]
      }
      frame "DB: Ventas" {
        n197 = Unbundle By Name(w433) -> ("DB"=w430:T3)
        n198 = call <vilib>:"DB Tools Select Data.vi"("error in (no error)"=w435, "table"="Ventas", "connection reference"=w430) -> ("error out"=w434:errorcluster, "data"=w428:variant[][], "connection reference out"=w431:T3)  [unwired: 3 in]
        n199 = Variant To Data(type=string[][] [] ("table"), Variant=w428) -> (data=w426:string[][])  [unwired: 1 in, 1 out]
        n200 = property on="Ventas" class="MCListbox (strict)"("ItemNames"=w426) -> ()  [unwired: 2 in, 2 out]
        n201 = Bundle By Name(cluster=w433, "DB"=w431, "Ventas"=w426) -> (w432:T4)
        n202 = call <vilib>:"Add State(s) to Queue__JKI_lib_State_Machine.vi"("State(s) in (\"\")"=w437) -> ("States Out"=w436:string)  [unwired: 14 in]
      }
      frame "DB: Add Venta" {
        n203 = Unbundle By Name(w452) -> ("Ventas"=w447:string[][], "DB"=w449:T3)
        n204 = property on="TOTAL" class="DigNum (strict)"() -> ("Value"=w444:dbl)  [unwired: 2 in, 2 out]
        n205 = Index Array(array=w447, index (col)=0 ("disabled index (col)")) -> (element=w445:string[])  [unwired: 1 in]
        n206 = Number To Decimal String(number=w444) -> (decimal integer string=w442:string)  [unwired: 1 in]
        n207 = property on="Orden" class="Str"() -> ("Value"=w443:string)  [unwired: 2 in, 2 out]
        n208 = Array Size(array=w445) -> (size(s)=w439:i32)
        n209 = Increment(x=w439) -> (x+1=w438:i32)
        n210 = Bundle(w438, "Value"=w443, w442) -> (w441:cluster{i32, "Value":string, string})  [unwired: 1 in]
        n211 = call <vilib>:"DB Tools Insert Data.vi"("data"=w441, "error in (no error)"=w454, "columns"=string[] ["ID", "Productos", "Total"], "table"="Ventas", "connection reference"=w449) -> ("error out"=w453:errorcluster, "connection reference out"=w450:T3)  [unwired: 5 in]
        n212 = Bundle By Name(cluster=w452, "DB"=w450) -> (w451:T4)
        n213 = call <vilib>:"Add State(s) to Queue__JKI_lib_State_Machine.vi"("State(s) in (\"\")"=w456) -> ("States Out"=w455:string)  [unwired: 14 in]
      }
      frame "Cambio" {
        n214 = property on="Tarjeta" class="Bool (strict)"() -> ("Value"=w457:bool)  [unwired: 2 in, 2 out]
        n215 = case shown="False" w457 {
          frame False {
            n216 = property on="Pesos" class="Bool (strict)"() -> ("Value"=w464:bool)  [unwired: 2 in, 2 out]
            n217 = property on="PAGO CON:" class="DigNum (strict)"() -> ("Value"=w463:dbl)  [unwired: 2 in, 2 out]
            n218 = case shown="False" w464 {
              tunnel: w463 -> [w472 w474]
              tunnel: [w473 w474] -> w462
              frame False {
                n219 = property on="Tipo de Cambio Dolares" class="DigNum (strict)"() -> ("Value"=w471:dbl)  [unwired: 2 in, 2 out]
                n220 = Multiply(x=w472, y=w471) -> (x*y=w473:dbl)
              }
              frame True {
              }
            }
            n221 = property on="TOTAL" class="DigNum (strict)"() -> ("Value"=w470:dbl)  [unwired: 2 in, 2 out]
            n222 = Subtract(x=w462, y=w470) -> (x-y=w468:dbl)
            n223 = Greater Than 0?(x=w468) -> (x > 0?=w469:bool)
            n224 = Less Than 0?(x=w468) -> (x < 0?=w467:bool)
            n225 = case shown="False" w469 {
              tunnel: w468 -> [w477 w484]
              tunnel: w467 -> [w478 _]
              tunnel: [w476 w484] -> w465
              tunnel: [w475 u32 6618880] -> w466
              frame False {
                n226 = case shown="False" w478 {
                  tunnel: [w480 w482] -> w476
                  tunnel: w477 -> [w480 w482]
                  tunnel: [u32 16777215 u32 16755872] -> w475
                  frame False {
                  }
                  frame True {
                  }
                }
              }
              frame True {
              }
            }
            n227 = property on="Cambio (Pesos)" class="DigNum (strict)"("NumText.BGColor"=w466, "Value"=w465) -> ()  [unwired: 2 in, 2 out]
          }
          frame True {
            n228 = property on="Cambio (Pesos)" class="DigNum (strict)"("NumText.BGColor"=u32 16777225, "Value"=0.0 ("Cambio")) -> ()  [unwired: 2 in, 2 out]
          }
        }
        n229 = call <vilib>:"Add State(s) to Queue__JKI_lib_State_Machine.vi"("State(s) in (\"\")"=w461) -> ("States Out"=w460:string)  [unwired: 14 in]
      }
    }
  }
